vi "shooter Controller.vi"(8 "error in":errorcluster) -> ()   [LabVIEW 2015]
doc: "This VI executes continuously carrying out the current operation and responding to updates or new operations. It will often contain the timing or control code that is difficult to place directly in TeleOp. This VI generally opens all sensors and motors and isolates the rest of the robot code from knowing how the operations are carried out."
uses:
  shooter Setpoints.ctl
  shooter Operations.ctl
  <vilib>/Rock Robotics/WPI/SafetyOutput/WPI_SafetyOutputConfigMenu.ctl
  <vilib>/Rock Robotics/WPI/Solenoid/WPI_SolenoidChannel.ctl
  <vilib>/Rock Robotics/WPI/Solenoid/WPI_SolenoidValue.ctl
  <vilib>/Rock Robotics/WPI/MotorControl/WPI_MotorControlOpenCANTalonSRX.vi
  <vilib>/Rock Robotics/WPI/Solenoid/WPI_SolenoidOpenDouble.vi
  <vilib>/Rock Robotics/WPI/Utilities/WPI_GetSetVariantRefNum.vi
  <vilib>/Rock Robotics/WPI/Solenoid/WPI_SolenoidSetEnum.vi
  <vilib>/Rock Robotics/Network Tables/NT Write Boolean.vi
panel:
  in  "target ripums":dbl
  out "Numeric":dbl
  out "Current\nCmd":string
  # "Tip: It may be helpful to observe inputs and sensor values.\nYou may also want to display tuning or debugging controls."
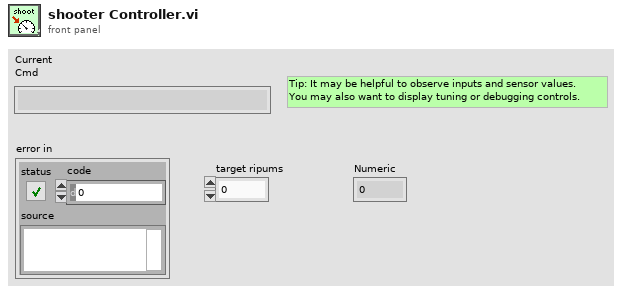
[diagram p1: front panel]
types:
  T1 = typedef "WPI_SolenoidChannel.ctl" = enum8{"Solenoid 0", "Solenoid 1", "Solenoid 2", "Solenoid 3", "Solenoid 4", "Solenoid 5", "Solenoid 6", "Solenoid 7", "Invalid"}
  T2 = typedef "WPI_SafetyOutputConfigMenu.ctl" = enum16{"Enable", "Disable"}
  T3 = typedef "shooter Setpoints.ctl" = cluster{"Operation":T4, "Setpoint":dbl, "Stop":dbl, "PID Angle Setpoint":dbl, "cowl on/off":dbl}
  T4 = typedef "shooter Operations.ctl" = enum16{"Reserve", "Read Current", "Immediate", "UpToSpeed", "MoveToAngle"}
  T5 = typedef "WPI_MotorControlDeviceRef.ctl" = cluster{"DeviceStatus":errorcluster, "Type":T6, "PWM":cluster{"PWM Channel":T7, "DeadBand":T8}, "CAN":cluster{"Device Number":u8, "Control Mode":T9, "Semaphore":T10, "Max Vout":dbl, "TalonSRX Control Mode":T11}, "Invert":bool}
  T6 = typedef "WPI_MotorControlType.ctl" = enum16{"PWM", "CAN", "CANTalonSRX"}
  T7 = typedef "FPGA_DIOPWMChannel.ctl" = enum8{"PWM 0", "PWM 1", "PWM 2", "PWM 3", "PWM 4", "PWM 5", "PWM 6", "PWM 7", "PWM 8", "PWM 9", "PWM MXP 0", "PWM MXP 1", "PWM MXP 2", "PWM MXP 3", "PWM MXP 4", "PWM MXP 5", "PWM MXP 6", "PWM MXP 7", "PWM MXP 8", "PWM MXP 9", "Invalid"}
  T8 = typedef "WPI_PWMDeadband.ctl" = cluster{"Name":string, "maxPositivePwm":i32, "minPositivePwm":i32, "centerPwm":i32, "maxNegativePwm":i32, "minNegativePwm":i32, "angularRange":u16}
  T9 = typedef "WPI_CANJaguar_ControlMode.ctl" = enum8{"Percent VBus", "Current", "Speed", "Position", "Voltage"}
  T10 = typedef "Semaphore RefNum" = refnum<k1>
  T11 = typedef "WPI_CANTalonSRX_APIControlMode.ctl" = enum8{"Percent VBus", "Speed", "Position", "Slave", "Unchanged / Invalid", "Voltage Compensation", "Current", "Motion Profile"}
  T12 = typedef "WPI_JoystickDevRef.ctl" = cluster{"Device":T13}
  T13 = typedef "WPI_JoystickDeviceEnum.ctl" = enum16{"USB 0", "USB 1", "USB 2", "USB 3", "USB 4", "USB 5"}
  T14 = typedef "WPI_SolenoidDevRef.ctl" = cluster{"DevStatus":errorcluster, "Pneumatics Control Module":u8, "Forward Solenoid Channel":T1, "Reverse Solenoid Channel":T1}
  T15 = typedef "Command Status Info.ctl" = cluster{"Name":string, "Status":T16, "notifier out":T17}
  T16 = typedef "Completion Status.ctl" = enum16{"Successful", "Aborted", "Incomplete"}
  T17 = typedef "Completion Notifier.ctl" = refnum<notifier>
  T18 = cluster{"Default Command":T3, "Command Timing":cluster{"Start Time (ms)":u32, "Iterations":i32}, "Command Arguments":cluster{"Command Info":T15, "Description":string, "Default Command":T3, "notifier out":refnum<notifier>, "Subsystem Name":string}}
  T19 = typedef "WPI_SolenoidValue.ctl" = enum16{"Off", "On", "Forward", "Reverse"}
  T20 = typedef "WPI_CANTalonSRX_GlobalStatus.ctl" = cluster{"Applied Throttle":dbl, "Module Enabled":bool, "CAN Error":errorcluster, "Closed Loop Error":dbl, "Forward Limit Switch Closed":bool, "Reverse Limit Switch Closed":bool, "Sensor Position":dbl, "Sensor Velocity":dbl, "Current":dbl, "Sticky Fault - Over Temp":bool, "Sticky Fault - Under Voltage":bool, "Sticky Fault - Forward Limit":bool, "Sticky Fault - Reverse Limit":bool, "Sticky Fault - Forward Soft Limit":bool, "Sticky Fault - Reverse Soft Limit":bool, "Brake is Enabled":bool, "Encoder Position":dbl, "Encoder Velocity":dbl, "Encoder Index Count":dbl, "Encoder A Pin State":bool, "Encoder B Pin State":bool, "Encoder Index Pin State":bool, "Analog In":dbl, "Analog In Velocity":dbl, "Temperature (C)":dbl, "Battery Voltage":dbl, "Control 5 Is Supported":bool, "Current Profile Slot Select":dbl, "Pos Div 8":bool, "Vel Div 4":bool, "Pulse Width Position":i32, "Pulse Width Velocity":i32, "Pulse Width Rise To Rise (us)":i32, "Pulse Width Rise To Fall (us)":i32, "Mot Prof Active Is Under Run":bool, "Mot Prof Active Has Under Run":bool, "Mot Prof Active Is Last":bool, "Mot Prof Active Velocity Only":bool, "Mot Prof Active Is Valid":bool, "Mot Prof Buffer Is Full":bool, "Mot Prof Active Profile Slot Select":i32, "Mot Prof NextID":i32, "Mot Prof Count":i32, "Mot Prof Active Velocity":dbl, "Mot Prof Active Position":dbl, "Mot Prof Output Enable":i32}
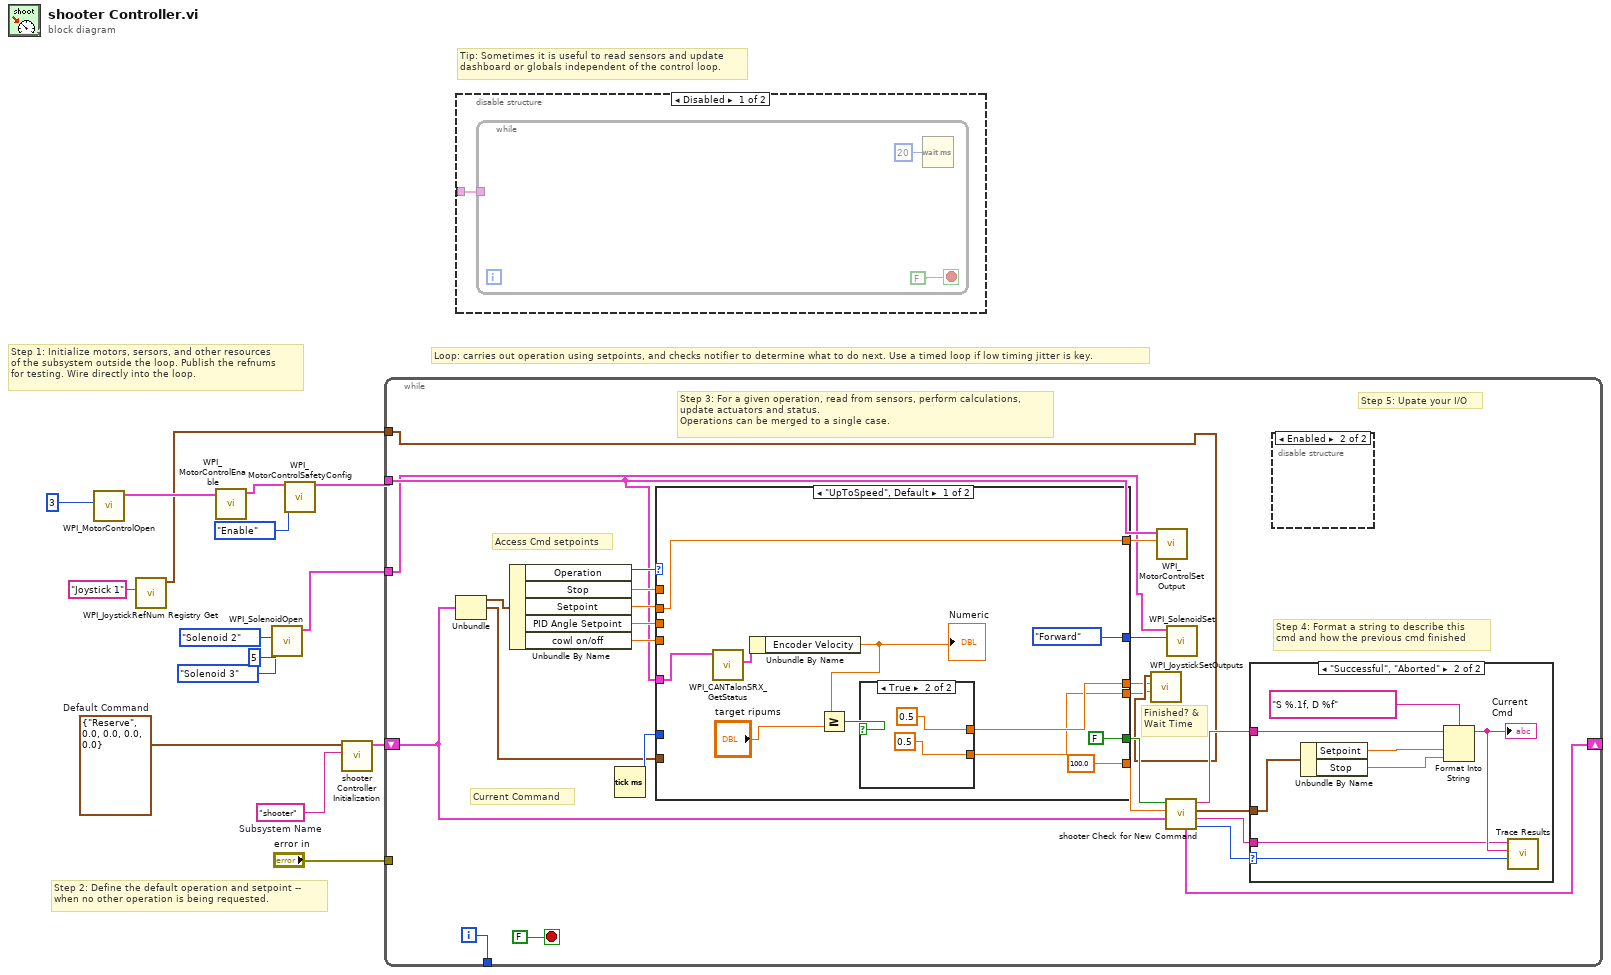
[diagram p0: block diagram]
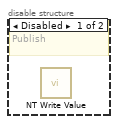
[diagram p3: hidden frame]
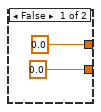
[diagram p5: hidden frame]
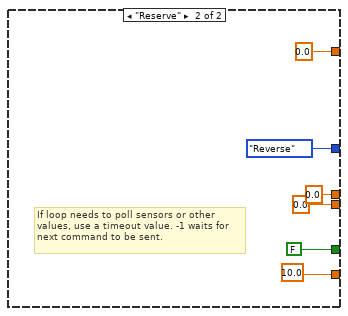
[diagram p6: hidden frame]
diagram:
  w12 = T3 {"Operation"=enum."Reserve", "Setpoint"=0.0, "Stop"=0.0, "PID Angle Setpoint"=0.0, "cowl on/off"=0.0}  # Default Command
  w13 = "shooter"  # Subsystem Name
  # "Tip: Sometimes it is useful to read sensors and update\ndashboard or globals independent of the control loop."
  # "Step 2: Define the default operation and setpoint --\nwhen no other operation is being requested."
  # "Step 1: Initialize motors, sersors, and other resources\nof the subsystem outside the loop. Publish the refnums\nfor testing. Wire directly into the loop."
  # "Loop: carries out operation using setpoints, and checks notifier to determine what to do next. Use a timed loop if low timing jitter is key."
  n1 = call-poly <vilib>:"WPI_MotorControlOpen.vi"("Device Number"=u8 3) -> ("MotorControlDeviceRef"=w10:T5)  [unwired: 9 in, 1 out]
  n2 = call <vilib>:"WPI_JoystickRefNum Registry Get.vi"("refnum name"="Joystick 1") -> ("JoystickDevRef"=w1:T12)  [unwired: 9 in, 1 out]
  n3 = call <vilib>:"WPI_MotorControlEnable.vi"("CAN MotorDevRef"=w10) -> ("CAN MotorDevRef"=w9:T5)  [unwired: 9 in, 1 out]
  n4 = call-poly <vilib>:"WPI_SolenoidOpen.vi"("Reverse Solenoid Channel"=WPI_SolenoidChannel."Solenoid 3", "Forward Solenoid Channel"=WPI_SolenoidChannel."Solenoid 2" ("Solenoid Channel"), "Pneumatics Control Module (0)"=u8 5) -> ("SolenoidDevRef"=w3:T14)  [unwired: 7 in, 1 out]
  n5 = call <vilib>:"WPI_MotorControlSafetyConfig.vi"("mode"=WPI_SafetyOutputConfigMenu."Enable", "MotorControlDevRef"=w9) -> ("MotorControlDevRef"=w7:T5)  [unwired: 8 in, 1 out]
  n6 = call "shooter Controller Initialization.vi"("Subsystem Name"=w13, "Default Command"=w12) -> ("Command Info"=w14:T18)  [unwired: 9 in]
  n7 = while {
    shift-right: [w31] -> _
    shift-left: w14 -> [w32]
    tunnel: [w39] -> _
    tunnel: "error in" -> [_]
    tunnel: w7 -> [w21]
    tunnel: w3 -> [w20]
    tunnel: w1 -> [w18]
    i -> [w39]
    stop <- FALSE stop-if-true
    # "Step 5: Upate your I/O"
    # "Step 4: Format a string to describe this\ncmd and how the previous cmd finished"
    # "Current Command"
    # "Access Cmd setpoints"
    # "Finished? &\nWait Time"
    # "Step 3: For a given operation, read from sensors, perform calculations,\nupdate actuators and status.\nOperations can be merged to a single case."
    n8 = Unbundle(w32) -> ("Default Command"=w38:T3, "Command Timing"=w34:cluster{"Start Time (ms)":u32, "Iterations":i32})  [unwired: 1 out]
    n9 = Unbundle By Name(w38) -> ("Operation"=w37:T4, "Stop"=w36:dbl, "Setpoint"=w33:dbl, "PID Angle Setpoint"=w23:dbl, "cowl on/off"=w22:dbl)
    n10 = Tick Count (ms)() -> (millisecond timer value=w35:u32)
    n11 = case shown="\"UpToSpeed\", Default" w37 {
      tunnel: [100.0 10.0] -> w29
      tunnel: [FALSE ("ignore previous (F)") FALSE ("ignore previous (F)")] -> w30
      tunnel: w34 -> [_ _]
      tunnel: w36 -> [_ _]
      tunnel: w35 -> [_ _]
      tunnel: w33 -> [w58 _]
      tunnel: [w58 0.0 ("Setpoint")] -> w24
      tunnel: w23 -> [_ _]
      tunnel: w22 -> [_ _]
      tunnel: w21 -> [w56 _]
      tunnel: [WPI_SolenoidValue."Forward" ("Value") WPI_SolenoidValue."Reverse" ("Value")] -> w19
      tunnel: [w50 sgl 0.0 ("Right Rumble")] -> w17
      tunnel: [w49 sgl 0.0 ("Left Rumble")] -> w16
      frame "UpToSpeed", Default {
        n12 = call <vilib>:"WPI_CANTalonSRX_GetStatus.vi"("CAN Talon SRX Ref"=w56) -> ("Talon SRX Status"=w55:T20)  [unwired: 8 in, 2 out]
        n13 = Unbundle By Name(w55) -> ("Encoder Velocity"=w52:dbl)
        "Numeric" <- w52
        n14 = Greater Or Equal?(x=w52, y="target ripums") -> (x >= y?=w51:bool)
        n15 = case shown="True" w51 {
          tunnel: [sgl 0.0 ("Right Rumble") sgl 0.5 ("Right Rumble")] -> w50
          tunnel: [sgl 0.0 ("Left Rumble") sgl 0.5 ("Left Rumble")] -> w49
          frame False {
          }
          frame True {
          }
        }
      }
      frame "Reserve" {
        # "If loop needs to poll sensors or other\nvalues, use a timeout value. -1 waits for\nnext command to be sent."
      }
    }
    n16 = call <vilib>:"WPI_JoystickSetOutputs.vi"("Right Rumble"=w16, "Left Rumble"=w17, "JoystickDevRef"=w18) -> ()  [unwired: 7 in, 2 out]
    n17 = call <vilib>:"WPI_MotorControlSetOutput.vi"("Output"=w24, "MotorControlDevRef"=w21) -> ()  [unwired: 7 in, 3 out]
    n18 = call "shooter Check for New Command.vi"("Current Command"=w32, "Wait time (ms)"=w29, "Finished?"=w30) -> ("Completion"=w25:T16, "Subsystem Name"=w26:string, "Current Command"=w27:T3, "Initial Trace String"=w28:string, "NextCommand"=w31:T18)  [unwired: 4 in]
    n19 = call-poly <vilib>:"WPI_SolenoidSet.vi"("Value"=w19, "SolenoidDevRef"=w20) -> ()  [unwired: 8 in, 2 out]
    n20 = case shown="\"Successful\", \"Aborted\"" w25 {
      selector: w25 -> [_ w48]
      tunnel: w28 -> [_ w44]
      tunnel: w27 -> [_ w45]
      tunnel: w26 -> [_ w41]
      frame "Incomplete", Default {
        # "Continuing current command"
      }
      frame "Successful", "Aborted" {
        # "Report and setup for next command"
        n21 = Unbundle By Name(w45) -> ("Setpoint"=w47:dbl, "Stop"=w42:dbl)
        n22 = Format Into String(format string="S %.1f, D %f", initial string=w44, w47, w42) -> (resulting string=w43:string)  [unwired: 1 in, 1 out]
        "Current\nCmd" <- w43
        n23 = call <vilib>:"Trace Results.vi"("Status of previous command"=w48, "Description"=w43, "Subsystem"=w41) -> ()  [unwired: 9 in]
      }
    }
    n24 = disable-structure shown="Enabled" {
      frame Disabled {
        # "Publish"
        n25 = call-poly <vilib>:"NT Write Value.vi"() -> ()  [unwired: 11 in, 1 out]
      }
      frame Enabled {
      }
    }
  }
  n26 = disable-structure shown="Disabled" {
    disable-tunnel: _ -> [w70 _]
    frame Disabled {
      n27 = while {
        tunnel: w70 -> [_]
        stop <- FALSE stop-if-true
        n28 = Wait (ms)(milliseconds to wait=u32 20) -> ()  [unwired: 1 out]
      }
    }
    frame Enabled {
    }
  }
